vi "DBL Speed to FXP.vi"(11 "Desired speed (RPM)":dbl min=0.0 format="%#_p") -> (0 "rpm max":dbl, 1 "rpm resolution":dbl, 2 "Actual speed (RPM)":dbl min=0.0 format="%#_p", 3 "FXP speed":fxp<+/-,23,2>, 4 "rpm min":dbl)   [LabVIEW 2015, in "Engine Simulation Toolkit Shared.lvlib"]
uses:
  Engine Simulation Toolkit Shared.lvlib
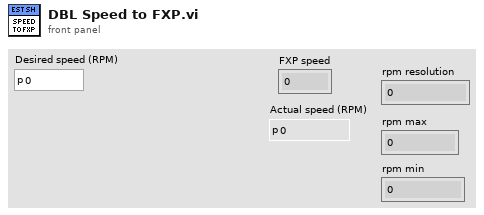
[diagram p1: front panel]
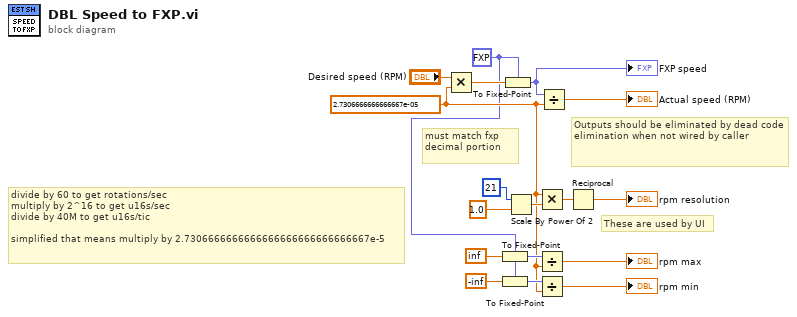
[diagram p0: block diagram]
diagram:
  w1 = fxp<+/-,23,2> 0.0
  w4 = 2.7306666666666667e-05 ("y")
  # "These are used by UI"
  # "must match fxp decimal portion"
  # "Outputs should be eliminated by dead code elimination when not wired by caller"
  # "divide by 60 to get rotations/sec\nmultiply by 2^16 to get u16s/sec\ndivide by 40M to get u16s/tic\n\nsimplified that means multiply by 2.7306666666666666666666666666667e-5"
  n1 = Multiply(x="Desired speed (RPM)", y=w4) -> (x*y=w15:dbl)
  n2 = To Fixed-Point(fixed-point type=w1, number=inf) -> (fixed-point=w6:fxp<+/-,23,2>)
  n3 = To Fixed-Point(fixed-point type=w1, number=-inf) -> (fixed-point=w5:fxp<+/-,23,2>)
  n4 = To Fixed-Point(fixed-point type=w1, number=w15) -> (fixed-point=w12:fxp<+/-,23,2>)
  "FXP speed" <- w12
  n5 = Scale By Power Of 2(n=i16 21, x=1.0) -> (x*2^n=w13:dbl)
  n6 = Multiply(x=w4, y=w13) -> (x*y=w11:dbl)
  n7 = Divide(x=w6, y=w4) -> (x/y=→"rpm max":dbl)
  n8 = Divide(x=w5, y=w4) -> (x/y=→"rpm min":dbl)
  n9 = Divide(x=w12, y=w4) -> (x/y=→"Actual speed (RPM)":dbl)
  n10 = Reciprocal(x=w11) -> (1/x=→"rpm resolution":dbl)
